vi "UpdateSpotMapSIMA.vi"(0 "Rawdata":T1, 1 "y":dbl[](array[numeric]), 2 "x":dbl[](array[numeric]), 5 "Mask (input)":T1, 9 "Display Input":T1, 11 "error in (no error)":errorcluster, 12 "radius":i32) -> (3 "Mask (output)":T1, 8 "Display (output":T1, 14 "error out":errorcluster)   [LabVIEW 2009]
uses:
  <vilib>/vision/Image Controls.llb/IMAQ Image.ctl
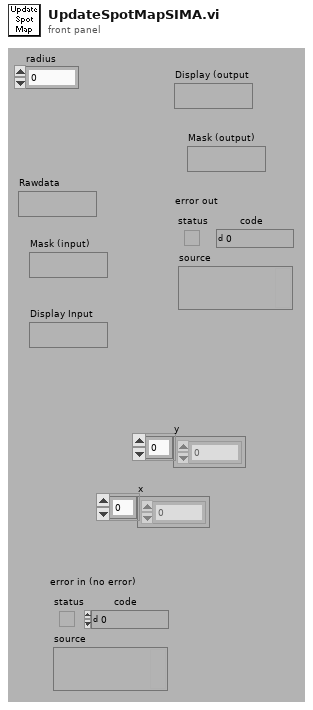
[diagram p1: front panel]
types:
  T1 = typedef "IMAQ Image.ctl" = refnum<image>
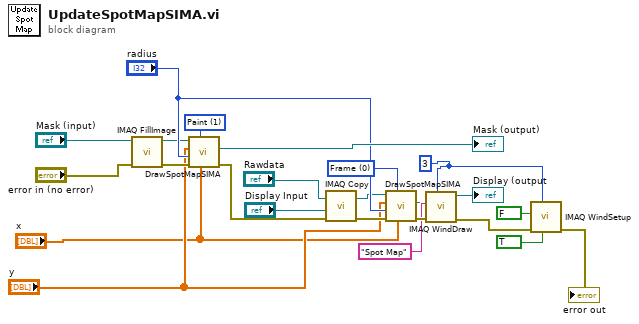
[diagram p0: block diagram]
diagram:
  w4 = 3 ("Window Number (0...15)")
  w13 = u16 1 items=["Frame", "Paint", "Invert Frame", "Invert Paint"] ("Draw Mode")
  w14 = u16 0 items=["Frame", "Paint", "Invert Frame", "Invert Paint"] ("Draw Mode")
  n1 = call "IMAQ FillImage"("error in (no error)"="error in (no error)", "Image"="Mask (input)") -> ("error out"=w20:errorcluster, "Image Out"=w21:T1)  [unwired: 8 in]
  n2 = call "DrawSpotMapSIMA.vi"("x"="x", "Draw Mode"=w13, "error in (no error)"=w20, "radius"="radius", "y"="y", "Image Dst"=w21) -> ("error out"=w11:errorcluster, "Spot Map"=→"Mask (output)":T1)  [unwired: 3 in]
  n3 = call "IMAQ Copy"("error in (no error)"=w11, "Image Dst"="Display Input", "Image Src"="Rawdata") -> ("error out"=w15:errorcluster, "Image Dst Out"=w3:T1)  [unwired: 3 in]
  n4 = call "DrawSpotMapSIMA.vi"("x"="x", "Draw Mode"=w14, "error in (no error)"=w15, "radius"="radius", "y"="y", "Image Dst"=w3) -> ("error out"=w17:errorcluster, "Spot Map"=w5:T1)  [unwired: 3 in]
  n5 = call "IMAQ WindDraw"("Window Number (0...15)"=w4, "error in (no error)"=w17, "Title"="Spot Map", "Image"=w5) -> ("error out"=w10:errorcluster, "Image Out (duplicate)"=→"Display (output":T1)  [unwired: 6 in]
  n6 = call "IMAQ WindSetup"("Window is floating? (No)"=TRUE, "Window Number (0...15)"=w4, "error in (no error)"=w10, "Window can close? (Yes)"=FALSE) -> ("error out"=→"error out":errorcluster)  [unwired: 7 in]
